vi "PCAProject.vi"(6 "Result in":dbl[][](array[numeric]), 8 "error in":errorcluster, 9 "EigenVectors":dbl[][](array[numeric]), 10 "Mean":dbl[][](array[numeric]), 11 "Data":dbl[][](array[numeric])) -> (0 "error out":errorcluster, 3 "Result out":dbl[][](array[numeric]))   [LabVIEW 2020, in "OpenLvVision_OpenCv.lvlib"]
doc: "Projects vector(s) to the principal component subspace."
uses:
  OpenLvVision_OpenCv.lvlib
  _LvHelpers/MatHandling/RegisterMat/RegisterMat_Array2D-DBL.vi
  _LvHelpers/MatHandling/ReadSize/ReadSizeMat_2DArray-DBL.vi
  _LvHelpers/MatHandling/WriteSize/WriteSizeMat_2DArray_DBL.vi
  Dlls/OlvOpenCvWrapper.dll
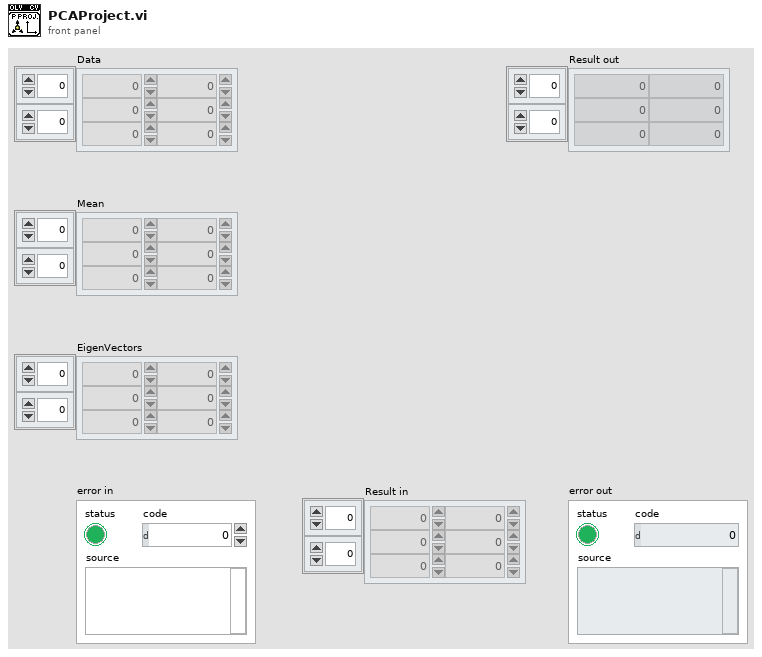
[diagram p1: front panel]
types:
  T1 = typedef "OpenLvVision_OpenCv.lvlib/MatInfo.ctl" = cluster{"Datatype":T2, "Height":i32, "Width":i32, "Channels":i32, "LineWidth":i32, "Null":u8}
  T2 = typedef "OpenLvVision_OpenCv.lvlib/LvDatatype.ctl" = enum32{"Undefined", "U8", "I8", "U16", "I16", "U32_Color", "I32", "U64_Color", "I64", "SGL", "DBL", "Complex SGL", "Complex DBL", "Array 1D U8", "Array 1D I8", "Array 1D U16", "Array 1D I16", "Array 1D U32_Color", "Array 1D I32", "Array 1D U64_Color", "Array 1D I64", "Array 1D SGL", "Array 1D DBL", "Array 1D Complex SGL", "Array 1D Complex DBL", "Array 2D U8", "Array 2D I8", "Array 2D U16", "Array 2D I16", "Array 2D U32", "Array 2D U32_Color", "Array 2D I32", "Array 2D U64", "Array 2D U64_Color", "Array 2D I64", "Array 2D SGL", "Array 2D DBL", "Array 2D Complex SGL", "Array 2D Complex DBL", "Image Mono U8", "Image Mono U16", "Image Mono I16", "Image Mono SGL", "Image Color U32", "Image Color U64", "ImageComplex Sgl", "Array1d_2dPointI32", "Array1d_2dPointSGL", "Array1d_2dPointDBL", "Array1d_3dPointI32", "Array1d_3dPointSGL", "Array1d_3dPointDBL", "Array1d_4dPointI32", "Array1d_4dPointSGL", "Array1d_4dPointDBL"}
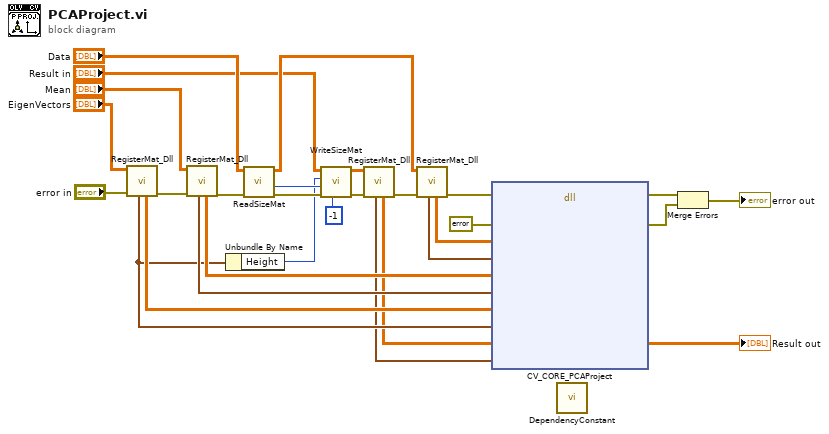
[diagram p0: block diagram]
diagram:
  n1 = call-poly "RegisterMat_Dll.vi"("error in"="error in", "Array in"="EigenVectors") -> ("error out"=w25:errorcluster, "AdressOrData"=w20:dbl[][], "Mat"=w18:T1)  [unwired: 6 in, 1 out]
  n2 = call-poly "RegisterMat_Dll.vi"("error in"=w25, "Array in"="Mean") -> ("error out"=w19:errorcluster, "AdressOrData"=w21:dbl[][], "Mat"=w22:T1)  [unwired: 6 in, 1 out]
  n3 = Unbundle By Name(w18) -> ("Height"=w7:i32)
  n4 = call-poly "ReadSizeMat.vi"("error in"=w19, "Array in"="Data") -> ("error out"=w10:errorcluster, "Height"=w8:i32, "Array out"=w13:dbl[][])  [unwired: 5 in, 2 out]
  n5 = call-poly "WriteSizeMat.vi"("Channel"=-1, "error in"=w10, "Height"=w8, "Width"=w7, "Array in"="Result in") -> ("error out"=w6:errorcluster, "Array out"=w3:dbl[][])  [unwired: 5 in]
  n6 = call-poly "RegisterMat_Dll.vi"("error in"=w6, "Array in"=w3) -> ("error out"=w5:errorcluster, "AdressOrData"=w2:dbl[][], "Mat"=w1:T1)  [unwired: 6 in, 1 out]
  n7 = call-poly "RegisterMat_Dll.vi"("error in"=w5, "Array in"=w13) -> ("error out"=w14:errorcluster, "AdressOrData"=w12:dbl[][], "Mat"=w11:T1)  [unwired: 6 in, 1 out]
  n8 = dll-call lib="C:/Users/lukas/Downloads/OpenLvVision_OpenCv/SourceCode/LabView/OpenLvVision_OpenCv/Dlls/OlvOpenCvWrapper.dll" fn="CV_CORE_PCAProject"(error in=w14, "Error"=errorcluster {"status"=FALSE, "code"=0, "source"=""} ("error constant"), "adressData"=w12, "matInfoData"=w11, "addressMean"=w21, "matInfoMean"=w22, "addressEigVec"=w20, "matInfoEigVec"=w18, "addressResult"=w2, "matInfoResult"=w1) -> (error out=w28:errorcluster, "Error"=w27:errorcluster, "addressResult"=→"Result out":dbl[][])  [unwired: 10 in, 1 out]
  n9 = call "DependencyConstant.vi"() -> ()  [unwired: 12 in]
  n10 = Merge Errors(w28, w27) -> (→"error out":errorcluster)
